vi "Change Switch Parameters.vi"(6 "NewAddress (\"\")":string="\"\"", 7 "NewType (0: ctSerial)":i32(ring) items=["ctSerial", "ctTCPIP"], 8 "error in (no error)":errorcluster, 9 "Address (\"\")":string="\"\"", 10 "Type (0: ctSerial)":i32(ring) items=["ctSerial", "ctTCPIP"], 11 "VISA resource name":refnum<visa-resource-name>) -> (0 "error out":errorcluster, 3 "VISA resource name out":refnum<visa-resource-name>)   [LabVIEW 2014, in "Stanford Research SR1.lvlib"]
doc: "Changes the communication parameters for the chain of switches at the original address to those specified by the NewType and NewAddress parameters."
uses:
  Stanford Research SR1.lvlib
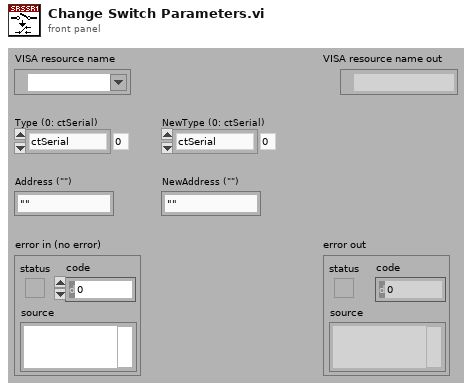
[diagram p1: front panel]
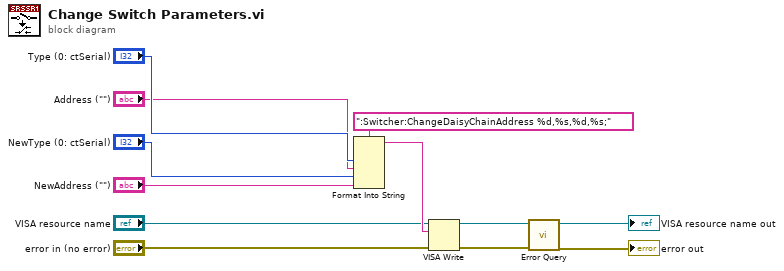
[diagram p0: block diagram]
diagram:
  n1 = Format Into String(format string=":Switcher:ChangeDaisyChainAddress %d,%s,%d,%s;", "Type (0: ctSerial)", "Address (\"\")", "NewType (0: ctSerial)", "NewAddress (\"\")") -> (resulting string=w7:string)  [unwired: 2 in, 1 out]
  n2 = VISA Write(VISA resource name="VISA resource name", write buffer=w7, error in (no error)="error in (no error)") -> (VISA resource name out=w4:refnum<visa-resource-name>, error out=w3:errorcluster)  [unwired: 1 out]
  n3 = call "Error Query.vi"("error in (no error)"=w3, "VISA resource name"=w4) -> ("error out"=→"error out":errorcluster, "VISA resource name out"=→"VISA resource name out":refnum<visa-resource-name>)  [unwired: 6 in, 2 out]
